vi "Test Generation.vi"(8 "error in (no error)":errorcluster) -> (0 "error out":errorcluster)   [LabVIEW 2020]
uses:
  78d0cb6d-c5d7-4722-b3c5-c800de6d1039.vi
  <vilib>/Analysis/baseanly.llb/Mean (DBL).vi
  b36c9cb4-86c7-423a-94e7-6ad977d17bf6.vi
  5950fcfc-c238-4952-ba95-fa3a390323ff.vi
  e736e450-6997-4243-b1af-984ee0668e3d.vi
  25f0c08c-bbd6-4d5e-a1e1-9ef245d2708f.vi
  a4779222-3a45-4624-a9fc-35823f218ceb.vi
  80d9f440-a25f-402f-9bd1-4821a057eb5e.vi
  <vilib>/numeric/Random Number (Range).vi
  <vilib>/numeric/Random Number (Range) U64.vi
  a4779222-3a45-4624-a9fc-35823f218ceb.vi/f460a025-ce12-4f10-b411-085793d100ac.vi
  <vilib>/numeric/sub_Random U32.vi
  <vilib>/addons/_JKI Toolkits/Caraya/classes/Assert/Assert Equal Value and Type_Variant.vi
  <vilib>/addons/_JKI Toolkits/Caraya/classes/Assert/Assert Almost Equal_Float.vi
  <vilib>/addons/_JKI Toolkits/Caraya/classes/Test/Test.lvclass
  <vilib>/addons/_JKI Toolkits/Caraya/classes/Assert/Assert.lvclass
  <vilib>/Analysis/NI_AALBase.lvlib
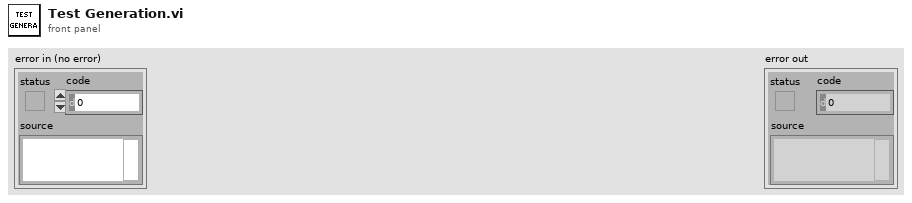
[diagram p1: front panel]
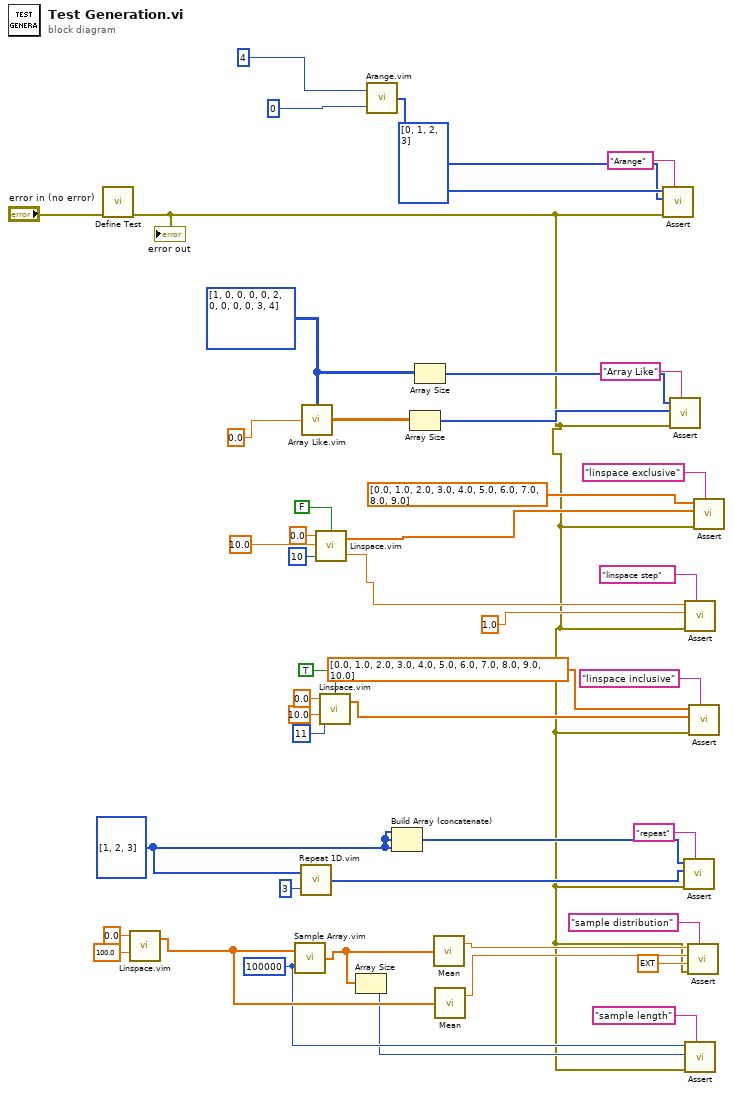
[diagram p0: block diagram]
diagram:
  w6 = 100000 ("N")
  w16 = i32[] [1, 2, 3]
  w40 = i32[][] [[1, 0, 0, 0], [0, 2, 0, 0], [0, 0, 3, 4]]
  n1 = call <vilib>:"Define Test.vi"("error in (no error)"="error in (no error)") -> ("error out"=w2:errorcluster)  [unwired: 10 in]
  "error out" <- w2
  n2 = call "Linspace.vim"("Stop"=100.0, "Start (Type)"=0.0) -> ("Values"=w11:dbl[])  [unwired: 2 in, 1 out]
  n3 = call "Sample Array.vim"("N"=w6, "Array"=w11) -> ("Samples"=w7:dbl[])
  n4 = call "Repeat 1D.vim"("Repeats"=u32 3, "Array"=w16) -> ("Repeated Array"=w17:i32[])
  n5 = call "Array Like.vim"("New Array Type & Default"=0.0, "Template Array"=w40) -> ("Initialized Array"=w39:dbl[][])
  n6 = call "Linspace.vim"("Include Endpoint (T)"=FALSE ("Include Endpoint"), "Num"=u32 10, "Stop"=10.0, "Start (Type)"=0.0) -> ("Step"=w29:dbl, "Values"=w30:dbl[])
  n7 = call "Linspace.vim"("Include Endpoint (T)"=TRUE ("Include Endpoint"), "Num"=u32 11, "Stop"=10.0, "Start (Type)"=0.0) -> ("Values"=w19:dbl[])  [unwired: 1 out]
  n8 = Array Size(array=w7) -> (size(s)=w5:i32)
  n9 = call "Arange.vim"("Low (Incl, type)"=0, "High (Excl)"=4) -> ("Array"=w44:i32[])  [unwired: 1 in]
  n10 = Build Array (concatenate)(w16, w16, w16) -> (w15:i32[])
  n11 = Array Size(array=w39) -> (size(s)=w37:i32[])
  n12 = Array Size(array=w40) -> (size(s)=w38:i32[])
  n13 = call-poly <vilib>:"Mean.vi"("X"=w7) -> ("mean"=w10:dbl)  [unwired: 1 out]
  n14 = call-poly <vilib>:"Mean.vi"("X"=w11) -> ("mean"=w9:dbl)  [unwired: 1 out]
  n15 = call-poly <vilib>:"Assert.vi"("Label"="Arange", "error in (no error)"=w2, "Y"=i32[] [0, 1, 2, 3] ("Array"), "X"=w44) -> ()  [unwired: 7 in, 1 out]
  n16 = call-poly <vilib>:"Assert.vi"("Label"="Array Like", "error in (no error)"=w2, "Y"=w37, "X"=w38) -> ()  [unwired: 7 in, 1 out]
  n17 = call-poly <vilib>:"Assert.vi"("Label"="repeat", "error in (no error)"=w2, "Y"=w17, "X"=w15) -> ()  [unwired: 7 in, 1 out]
  n18 = call-poly <vilib>:"Assert.vi"("Label"="linspace step", "error in (no error)"=w2, "Y"=1.0 ("Step"), "X"=w29) -> ()  [unwired: 7 in, 1 out]
  n19 = call-poly <vilib>:"Assert.vi"("Label"="sample length", "error in (no error)"=w2, "Y"=w5, "X"=w6) -> ()  [unwired: 7 in, 1 out]
  n20 = call-poly <vilib>:"Assert.vi"("Label"="sample distribution", "error in (no error)"=w2, "Tolerance"=ext 0.5, "Y"=w9, "X"=w10) -> ()  [unwired: 6 in, 1 out]
  n21 = call-poly <vilib>:"Assert.vi"("Label"="linspace inclusive", "error in (no error)"=w2, "Y"=w19, "X"=dbl[] [0.0, 1.0, 2.0, 3.0, 4.0, 5.0, 6.0, 7.0, 8.0, 9.0, 10.0] ("Values")) -> ()  [unwired: 7 in, 1 out]
  n22 = call-poly <vilib>:"Assert.vi"("Label"="linspace exclusive", "error in (no error)"=w2, "Y"=w30, "X"=dbl[] [0.0, 1.0, 2.0, 3.0, 4.0, 5.0, 6.0, 7.0, 8.0, 9.0] ("Values")) -> ()  [unwired: 7 in, 1 out]
